vi "Initialize.vi"(8 "error in":errorcluster, 11 "DMA in":refnum<class "DMA.lvclass">) -> (0 "error out":errorcluster, 3 "DMA out":refnum<class "DMA.lvclass">)   [LabVIEW 2015, in "DMA.lvclass"]
uses:
  DMA.lvclass
  Atmospheric/Gas Properties/Children/Air/Air.lvclass
  Particle Class/Particle Properties.lvclass
  Particle Class/Particle Properties.lvclass/Particle Properties.ctl
  DMA.lvclass/DMA.ctl
  Accessors/Write Particle.vi
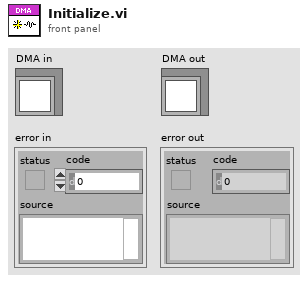
[diagram p1: front panel]
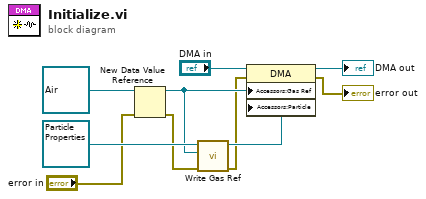
[diagram p0: block diagram]
diagram:
  n1 = New Data Value Reference(data value=refnum<class "Air.lvclass"> refnum ("Air"), error in="error in") -> (data value reference=w6:refnum<data-value>, error out=w4:errorcluster)
  n2 = call "Write Gas Ref.vi"("error in"=w4, "Gas Ref"=w6, "Particle Properties in"=refnum<class "Particle Properties.lvclass"> refnum ("Particles")) -> ("error out"=w3:errorcluster, "Particle Properties out"=w5:refnum<class "Particle Properties.lvclass">)  [unwired: 7 in]
  n3 = property class="DMA"(reference="DMA in", error in=w3, "Accessors:Gas Ref"=w6, "Accessors:Particle"=w5) -> (reference out=→"DMA out":refnum<class "DMA.lvclass">, error out=→"error out":errorcluster)
